vi "SEK2020v1VI10IrParaExtremidadePreta.vi"() -> ()   [LabVIEW 2016]
uses:
  <vilib>/NXT/Subs/LVHSConnector.ctl
  <vilib>/NXT/LegoClasses/BrickReference/BrickReference.lvclass
  <vilib>/NXT/Block Support/NXT_OutputPort.ctl
  <vilib>/NXT/Block Support/NXT_InputPort.ctl
  <vilib>/NXT/Dual Mode Library/Sensors/EV3_Color_Reflect.vi
  <vilib>/NXT/NXTIO Xnodes/NXTIONodeSubVIs/NXTStopMotors.vi
  <vilib>/NXT/NXTIO Xnodes/NXTIONodeSubVIs/NXTMoveMotors.vi
  <vilib>/NXT/Dual Mode Library/Waits/Wait_Num.vi
  <vilib>/NXT/NXTIO Xnodes/AddressXNode/NXTIOAddress.xnode
  <vilib>/NXT/NXTIO Xnodes/NXTIOXNode/NXTIO.xnode
panel:
  in  "Parâmetros":T1={"Azul Max EV3 Cor"=17, "Azul Min EV3 Cor"=0, "Verde Max EV3 Cor"=6, "Verde Min EV3 Cor"=0, "Vermelho Max Ev3 Cor"=0, "Vermelho Min EV3 Cor"=0, "Chão EV3 Cor"=0.0, "Branco Max EV3 Cor"=0.0, "Branco Min EV3 Cor"=0.0, "Preto Max EV3 Cor"=0.0, "Preto Min EV3 Cor"=0.0, "Distância Tubulação"=0.0, "Distância Frontal"=0.0, "Amarelo Max EV3 Cor"=0.0, "Amarelo Min EV3 Cor"=0.0, "Distância Lateral"=0.0, "90°"=0.0, "180°"=0.0, "Seguidor de Linha"=0.0}
  out "NXT/EV3 2":T2
  in  "NXT/EV3":T2
  # "Sensor EV3 Cor"
  # "Sensor Ultrassônico"
  # "Sensor Giroscópio"
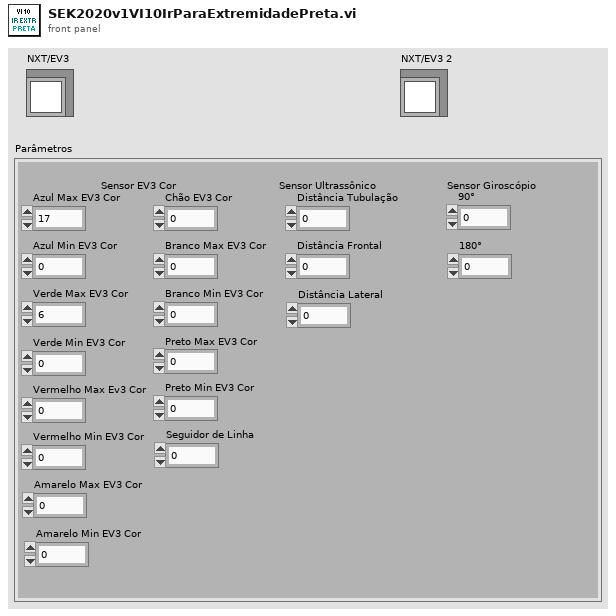
[diagram p1: front panel]
types:
  T1 = cluster{"Azul Max EV3 Cor":i32, "Azul Min EV3 Cor":i32, "Verde Max EV3 Cor":i32, "Verde Min EV3 Cor":i32, "Vermelho Max Ev3 Cor":i32, "Vermelho Min EV3 Cor":i32, "Chão EV3 Cor":sgl, "Branco Max EV3 Cor":sgl, "Branco Min EV3 Cor":sgl, "Preto Max EV3 Cor":sgl, "Preto Min EV3 Cor":sgl, "Distância Tubulação":sgl, "Distância Frontal":sgl, "Amarelo Max EV3 Cor":dbl, "Amarelo Min EV3 Cor":dbl, "Distância Lateral":sgl, "90°":sgl, "180°":sgl, "Seguidor de Linha":dbl}
  T2 = typedef "LVHSConnector.ctl" = refnum<class "BrickReference.lvclass">
  T3 = typedef "NXT_InputPort.ctl" = u32
  T4 = typedef "NXT_OutputPort.ctl" = u8
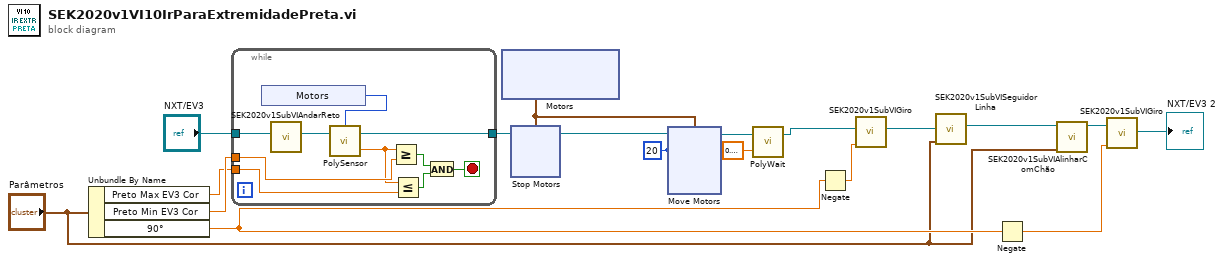
[diagram p0: block diagram]
diagram:
  w9 = i8 20 ("Power/Speed 1")
  n1 = Unbundle By Name("Parâmetros") -> ("Preto Max EV3 Cor"=w16:sgl, "Preto Min EV3 Cor"=w17:sgl, "90°"=w5:sgl)
  n2 = while {
    tunnel: "NXT/EV3" -> [w28]
    tunnel: w17 -> [w24]
    tunnel: w16 -> [w23]
    tunnel: [w20] -> w12
    stop <- w27 stop-if-true
    n3 = xnode "Motors"() -> ("Sensor"=w19:T3)
    n4 = call "SEK2020v1SubVIAndarReto.vi"("NXT/EV3"=w28) -> ("NXT/EV3 2"=w21:T2)  [unwired: 9 in]
    n5 = call-poly <vilib>:"PolySensor.vi"("NXT/EV3"=w21, "Port (Port 1)"=w19) -> ("Scaled Value"=w22:sgl, "NXT/EV3"=w20:T2)  [unwired: 1 in]
    n6 = Greater Or Equal?(x=w22, y=w24) -> (x >= y?=w25:bool)
    n7 = Less Or Equal?(x=w22, y=w23) -> (x <= y?=w26:bool)
    n8 = And(x=w25, y=w26) -> (x .and. y?=w27:bool)
  }
  n9 = xnode "Motors"() -> ("Motor"=w10:cluster{"Port":T4, "Port":T4})
  n10 = xnode "Stop Motors"("Motors"=w10, "NXT/EV3"=w12) -> ("NXT/EV3"=w11:T2)
  n11 = xnode "Move Motors"("Power/Speed 2"=w9, "Power/Speed 1"=w9, "Motors"=w10, "NXT/EV3"=w11) -> ("NXT/EV3"=w8:T2)
  n12 = call-poly <vilib>:"PolyWait.vi"("Time (1 sec)"=sgl 0.3, "NXT/EV3"=w8) -> ("NXT/EV3"=w7:T2)  [unwired: 2 in]
  n13 = Negate(x=w5) -> (-x=w13:sgl)
  n14 = call "SEK2020v1SubVIGiro.vi"("ANGULO"=w13, "NXT/EV3"=w7) -> ("NXT/EV3 2"=w3:T2)  [unwired: 7 in]
  n15 = call "SEK2020v1SubVISeguidorLinha.vi"("Parâmetros"="Parâmetros", "NXT/EV3"=w3) -> ("NXT/EV3 3"=w2:T2)  [unwired: 9 in]
  n16 = Negate(x=w5) -> (-x=w4:sgl)
  n17 = call "SEK2020v1SubVIAlinharComChão.vi"("Parâmetros"="Parâmetros", "NXT/EV3"=w2) -> ("NXT/EV3 2"=w15:T2)  [unwired: 9 in]
  n18 = call "SEK2020v1SubVIGiro.vi"("ANGULO"=w4, "NXT/EV3"=w15) -> ("NXT/EV3 2"=→"NXT/EV3 2":T2)  [unwired: 7 in]
